vi "unified-2CAM.VI"() -> ()   [LabVIEW 2015]
uses:
  board.vis/Globals.vi
  <vilib>/Analysis/NI_AALBase.lvlib
panel:
  in  "send all":bool
  in  "Offset ADC 8":u16=49000
  in  "Offset ADC 3":u16=49000
  in  "Offset ADC 7":u16=49000
  in  "Offset ADC 2":u16=49000
  in  "Offset ADC 6":u16=49000
  in  "Offset ADC 1":u16=49000
  in  "Offset ADC 5":u16=49000
  in  "Offset ADC 4":u16=49000
  in  "custom pattern: 14bits (hex)":fxp<+,14,14>=100.0 format="%x"
  out "data adr  0x25":u16 format="%x"
  out "data adr  0x26":u16 format="%x"
  out "custom pattern: 14bits (dec)":fxp<+,14,14>
  in  "ADC mode":enum32{"1", "2", "3"}(radio)=enum."3"
  out "Signalverlaufgraph Cam 2":u16[](graph)=[100, 100, 100, 100, 100, 100, 100, 100, 100, 100, 100, 100, 100, 100, 100, 100, 100, 100, 100, 100, 100, 100, 100, 100, 100, 100, 100, 100, 100, 100, 100, 100, 100, 100, 100, 100, 100, 100, 100, 100, 100, 100, 100, 100, 100, 100, 100, 100, 100, 100, 100, 100, 100, 100, 100, 100, 100, 100, 100, 100, 100, 100, 100, 100, 100, 100, 100, 100, 100, 100, 100, 100, 100, 100, 100, 100, 100, 100, 100, 100, 100, 100, 100, 100, 100, 100, 100, 100, 100, 100, 100, 100, 100, 100, 100, 100, 100, 100, 100, 100, 100, 100, 100, 100, 100, 100, 100, 100, 100, 100, 100, 100, 100, 100, 100, 100, 100, 100, 100, 100, 100, 100, 100, 100, 100, 100, 100, 100, 100, 100, 100, 100, 100, 100, 100, 100, 100, 100, 100, 100, 100, 100, 100, 100, 100, 100, 100, 100, 100, 100, 100, 100, 100, 100, 100, 100, 100, 100, 100, 100, 100, 100, 100, 100, 100, 100, 100, 100, 100, 100, 100, 100, 100, 100, 100, 100, 100, 100, 100, 100, 100, 100, 100, 100, 100, 100, 100, 100, 100, 100, 100, 100, 100, 100, 100, 100, 100, 100, 100, 100, 100, 100, 100, 100, 100, 100, 100, 100, 100, 100, 100, 100, 100, 100, 100, 100, 100, 100, 100, 100, 100, 100, 100, 100, 100, 100, 100, 100, 100, 100, 100, 100, 100, 100, 100, 100, 100, 100, 100, 100, 100, 100, 100, 100, 100, 100, 100, 100, 100, 100, 100, 100, 100, 100, 100, 100, 100, 100, 100, 100, 100, 100, 100, 100, 100, 100, 100, 100, 100, 100, 100, 100, 100, 100, 100, 100, 100, 100, 100, 100, 100, 100, 100, 100, 100, 100, 100, 100, 100, 100, 100, 100, 100, 100, 100, 100, 100, 100, 100, 100, 100, 100, 100, 100, 100, 100, 100, 100, 100, 100, 100, 100, 100, 100, 100, 100, 100, 100, 100, 100, 100, 100, 100, 100, 100, 100, 100, 100, 100, 100, 100, 100, 100, 100, 100, 100, 100, 100, 100, 100, 100, 100, 100, 100, 100, 100, 100, 100, 100, 100, 100, 100, 100, 100, 100, 100, 100, 100, 100, 100, 100, 100, 100, 100, 100, 100, 100, 100, 100, 100, 100, 100, 100, 100, 100, 100, 100, 100, 100, 100, 100, 100, 100, 100, 100, 100, 100, 100, 100, 100, 100, 100, 100, 100, 100, 100, 100, 100, 100, 100, 100, 100, 100, 100, 100, 100, 100, 100, 100, 100, 100, 100, 100, 100, 100, 100, 100, 100, 100, 100, 100, 100, 100, 100, 100, 100, 100, 100, 100, 100, 100, 100, 100, 100, 100, 100, 100, 100, 100, 100, 100, 100, 100, 100, 100, 100, 100, 100, 100, 100, 100, 100, 100, 100, 100, 100, 100, 100, 100, 100, 100, 100, 100, 100, 100, 100, 100, 100, 100, 100, 100, 100, 100, 100, 100, 100, 100, 100, 100, 100, 100, 100, 100, 100, 100, 100, 100, 100, 100, 100, 100, 100, 100, 100, 100, 100, 100, 100, 100, 100, 100, 100, 100, 100, 100, 100, 100, 100, 100, 100, 100, 100, 100, 100, 100, 100, 100, 100, 100, 100, 100, 100, 100, 100, 100, 100, 100, 100, 100, 100, 100, 100, 100, 100, 100, 100, 100, 100, 100, 100, 100, 100, 100, 100, 100, 100, 100, 100, 100, 100, 100, 100, 100, 100, 100, 100, 100, 100, 100, 100, 100, 100, 100, 100, 100, 100, 100, 100, 100, 100, 100, 100, 100, 100, 100, 100, 100, 100, 100, 100, 100, 100, 100, 100, 100, 100, 100, 100, 100, 100, 100, 100, 100, 100, 100, 100, 100, 100, 100, 100, 100, 100, 100, 100, 100, 100, 100, 100, 100, 100, 100, 100, 100, 100, 100, 100, 100, 100, 100, 100, 100, 100, 100, 100, 100, 100, 100, 100, 100, 100, 100, 100, 100, 100, 100, 100, 100, 100, 100, 100, 100, 100, 100, 100, 100, 100, 100, 100, 100, 100, 100, 100, 100, 100, 100, 100, 100, 100, 100, 100, 100, 100, 100, 100, 100, 100, 100, 100, 100, 100, 100, 100, 100, 100, 100, 100, 100, 100, 100, 100, 100, 100, 100, 100, 100, 100, 100, 100, 100, 100, 100, 100, 100, 100, 100, 100, 100, 100, 100, 100, 100, 100, 100, 100, 100, 100, 100, 100, 100, 100, 100, 100, 100, 100, 100, 100, 100, 100, 100, 100, 100, 100, 100, 100, 100, 100, 100, 100, 100, 100, 100, 100, 100, 100, 100, 100, 100, 100, 100, 100, 100, 100, 100, 100, 100, 100, 100, 100, 100, 100, 100, 100, 100, 100, 100, 100, 100, 100, 100, 100, 100, 100, 100, 100, 100, 100, 100, 100, 100, 100, 100, 100, 100, 100, 100, 100, 100, 100, 100, 100, 100, 100, 100, 100, 100, 100, 100, 100, 100, 100, 100, 100, 100, 100, 100, 100, 100, 100, 100, 100, 100, 100, 100, 100, 100, 100, 100, 100, 100, 100, 100, 100, 100, 100, 100, 100, 100, 100, 100, 100, 100, 100, 100, 100, 100, 100, 100, 100, 100, 100, 100, 100, 100, 100, 100, 100, 100, 100, 100, 100, 100, 100, 100, 100, 100, 100, 100, 100, 100, 100, 100, 100, 100, 100, 100, 100, 100, 100, 100, 100, 100, 100, 100, 100, 100, 100, 100, 100, 100, 100, 100, 100, 100, 100, 100, 100, 100, 100, 100, 100, 100, 100, 100, 100, 100, 100, 100, 100, 100, 100, 100, 100, 100, 100, 100, 100, 100, 100, 100, 100, 100, 100, 100, 100, 100, 100, 100, 100, 100, 100, 100, 100, 100, 100, 100, 100, 100, 100, 100, 100, 100, 100, 100, 100, 100, 100, 100, 100, 100, 100, 100, 100, 100, 100, 100, 100, 100, 100, 100, 100, 100, 100, 100, 100, 100, 100, 100, 100, 100, 100, 100, 100, 100, 100, 100, 100, 100, 100, 100, 100, 100, 100, 100, 100, 100, 100, 100, 100, 100, 100, 100, 100, 100, 100, 100, 100, 100, 100, 100, 100, 100, 100, 100, 100, 100, 100, 100, 100, 100, 100, 100, 100, 100, 100, 100, 100, 100, 100, 100, 100, 100, 100, 100, 100, 100, 100, 100, 100, 100, 100, 100, 100, 100, 100, 100, 100, 100, 100, 100, 100, 100, 100, 100, 100, 100, 100, 100, 100, 100, 100, 100, 100, 100, 100, 100, 100, 100, 100, 100, 100, 100, 100, 100, 100, 100, 100, 100, 100, 100, 100, 100, 100, 100, 100, 100, 100, 100, 100, 100, 100, 100, 100, 100, 100, 100, 100, 100, 100, 100, 100, 100, 100, 100, 100, 100, 100, 100, 100, 100, 100, 100, 100, 100, 100, 100, 100, 100, 100]
  in  "extTrig":bool
  in  "ext. trig. slope":enum32{"1", "2", "3"}(radio)
  out "tRMS":dbl format="%0#.1f"
  out "mean":dbl=100.0 format="%#_4f"
  in  "rms_pixel":u16=100
  in  "is FFT":bool=TRUE
  in  "IR gain":bool
  in  "continuous":bool
  out "curr.block":u8=4
  out "Measure ON":bool
  in  "Board select\n1: board 1\n2: board 2\n3: both boards":u8=3
  in  "no.of blocks (nob)\npress enter":u32=4
  in  "block":u32(slide)=2 max=10 scale=0.9..4.0
  out "Signalverlaufgraph Board 2":u16[](graph)=[0, 0, 543, 543, 0, 1, 0, 0, 2, 2, 3, 3, 4, 4, 5, 5, 6, 6, 7, 7, 8, 8, 9, 9, 10, 10, 11, 11, 12, 12, 13, 13, 14, 14, 15, 15, 16, 16, 17, 17, 18, 18, 19, 19, 20, 20, 21, 21, 22, 22, 23, 23, 24, 24, 25, 25, 26, 26, 27, 27, 28, 28, 29, 29, 30, 30, 31, 31, 32, 32, 33, 33, 34, 34, 35, 35, 36, 36, 37, 37, 38, 38, 39, 39, 40, 40, 41, 41, 42, 42, 43, 43, 44, 44, 45, 45, 46, 46, 47, 47, 48, 48, 49, 49, 50, 50, 51, 51, 52, 52, 53, 53, 54, 54, 55, 55, 56, 56, 57, 57, 58, 58, 59, 59, 60, 60, 61, 61, 62, 62, 63, 63, 64, 64, 65, 65, 66, 66, 67, 67, 68, 68, 69, 69, 70, 70, 71, 71, 72, 72, 73, 73, 74, 74, 75, 75, 76, 76, 77, 77, 78, 78, 79, 79, 80, 80, 81, 81, 82, 82, 83, 83, 84, 84, 85, 85, 86, 86, 87, 87, 88, 88, 89, 89, 90, 90, 91, 91, 92, 92, 93, 93, 94, 94, 95, 95, 96, 96, 97, 97, 98, 98, 99, 99, 100, 100, 101, 101, 102, 102, 103, 103, 104, 104, 105, 105, 106, 106, 107, 107, 108, 108, 109, 109, 110, 110, 111, 111, 112, 112, 113, 113, 114, 114, 115, 115, 116, 116, 117, 117, 118, 118, 119, 119, 120, 120, 121, 121, 122, 122, 123, 123, 124, 124, 125, 125, 126, 126, 127, 127, 128, 128, 129, 129, 130, 130, 131, 131, 132, 132, 133, 133, 134, 134, 135, 135, 136, 136, 137, 137, 138, 138, 139, 139, 140, 140, 141, 141, 142, 142, 143, 143, 144, 144, 145, 145, 146, 146, 147, 147, 148, 148, 149, 149, 150, 150, 151, 151, 152, 152, 153, 153, 154, 154, 155, 155, 156, 156, 157, 157, 158, 158, 159, 159, 160, 160, 161, 161, 162, 162, 163, 163, 164, 164, 165, 165, 166, 166, 167, 167, 168, 168, 169, 169, 170, 170, 171, 171, 172, 172, 173, 173, 174, 174, 175, 175, 176, 176, 177, 177, 178, 178, 179, 179, 180, 180, 181, 181, 182, 182, 183, 183, 184, 184, 185, 185, 186, 186, 187, 187, 188, 188, 189, 189, 190, 190, 191, 191, 192, 192, 193, 193, 194, 194, 195, 195, 196, 196, 197, 197, 198, 198, 199, 199, 200, 200, 201, 201, 202, 202, 203, 203, 204, 204, 205, 205, 206, 206, 207, 207, 208, 208, 209, 209, 210, 210, 211, 211, 212, 212, 213, 213, 214, 214, 215, 215, 216, 216, 217, 217, 218, 218, 219, 219, 220, 220, 221, 221, 222, 222, 223, 223, 224, 224, 225, 225, 226, 226, 227, 227, 228, 228, 229, 229, 230, 230, 231, 231, 232, 232, 233, 233, 234, 234, 235, 235, 236, 236, 237, 237, 238, 238, 239, 239, 240, 240, 241, 241, 242, 242, 243, 243, 244, 244, 245, 245, 246, 246, 247, 247, 248, 248, 249, 249, 250, 250, 251, 251, 252, 252, 253, 253, 254, 254, 255, 255, 256, 256, 257, 257, 258, 258, 259, 259, 260, 260, 261, 261, 262, 262, 263, 263, 264, 264, 265, 265, 266, 266, 267, 267, 268, 268, 269, 269, 270, 270, 271, 271, 272, 272, 273, 273, 274, 274, 275, 275, 276, 276, 277, 277, 278, 278, 279, 279, 280, 280, 281, 281, 282, 282, 283, 283, 284, 284, 285, 285, 286, 286, 287, 287, 288, 288, 289, 289, 290, 290, 291, 291, 292, 292, 293, 293, 294, 294, 295, 295, 296, 296, 297, 297, 298, 298, 299, 299, 300, 300, 301, 301, 302, 302, 303, 303, 304, 304, 305, 305, 306, 306, 307, 307, 308, 308, 309, 309, 310, 310, 311, 311, 312, 312, 313, 313, 314, 314, 315, 315, 316, 316, 317, 317, 318, 318, 319, 319, 320, 320, 321, 321, 322, 322, 323, 323, 324, 324, 325, 325, 326, 326, 327, 327, 328, 328, 329, 329, 330, 330, 331, 331, 332, 332, 333, 333, 334, 334, 335, 335, 336, 336, 337, 337, 338, 338, 339, 339, 340, 340, 341, 341, 342, 342, 343, 343, 344, 344, 345, 345, 346, 346, 347, 347, 348, 348, 349, 349, 350, 350, 351, 351, 352, 352, 353, 353, 354, 354, 355, 355, 356, 356, 357, 357, 358, 358, 359, 359, 360, 360, 361, 361, 362, 362, 363, 363, 364, 364, 365, 365, 366, 366, 367, 367, 368, 368, 369, 369, 370, 370, 371, 371, 372, 372, 373, 373, 374, 374, 375, 375, 376, 376, 377, 377, 378, 378, 379, 379, 380, 380, 381, 381, 382, 382, 383, 383, 384, 384, 385, 385, 386, 386, 387, 387, 388, 388, 389, 389, 390, 390, 391, 391, 392, 392, 393, 393, 394, 394, 395, 395, 396, 396, 397, 397, 398, 398, 399, 399, 400, 400, 401, 401, 402, 402, 403, 403, 404, 404, 405, 405, 406, 406, 407, 407, 408, 408, 409, 409, 410, 410, 411, 411, 412, 412, 413, 413, 414, 414, 415, 415, 416, 416, 417, 417, 418, 418, 419, 419, 420, 420, 421, 421, 422, 422, 423, 423, 424, 424, 425, 425, 426, 426, 427, 427, 428, 428, 429, 429, 430, 430, 431, 431, 432, 432, 433, 433, 434, 434, 435, 435, 436, 436, 437, 437, 438, 438, 439, 439, 440, 440, 441, 441, 442, 442, 443, 443, 444, 444, 445, 445, 446, 446, 447, 447, 448, 448, 449, 449, 450, 450, 451, 451, 452, 452, 453, 453, 454, 454, 455, 455, 456, 456, 457, 457, 458, 458, 459, 459, 460, 460, 461, 461, 462, 462, 463, 463, 464, 464, 465, 465, 466, 466, 467, 467, 468, 468, 469, 469, 470, 470, 471, 471, 472, 472, 473, 473, 474, 474, 475, 475, 476, 476, 477, 477, 478, 478, 479, 479, 480, 480, 481, 481, 482, 482, 483, 483, 484, 484, 485, 485, 486, 486, 487, 487, 488, 488, 489, 489, 490, 490, 491, 491, 492, 492, 493, 493, 494, 494, 495, 495, 496, 496, 497, 497, 498, 498, 499, 499, 500, 500, 501, 501, 502, 502, 503, 503, 504, 504, 505, 505, 506, 506, 507, 507, 508, 508, 509, 509, 510, 510, 511, 511, 512, 512, 513, 513, 514, 514, 515, 515, 516, 516, 517, 517, 518, 518, 519, 519, 520, 520, 521, 521, 522, 522, 523, 523, 524, 524, 525, 525, 526, 526, 527, 527, 528, 528, 529, 529, 530, 530, 531, 531, 532, 532, 533, 533, 534, 534, 535, 535, 536, 536, 537, 537, 538, 538, 539, 539, 540, 540, 541, 541]
  out "Signalverlaufgraph":u16[](graph)=[542, 542, 543, 543, 49152, 2, 0, 566, 2, 2, 3, 3, 4, 4, 5, 5, 6, 6, 7, 7, 8, 8, 9, 9, 10, 10, 11, 11, 12, 12, 13, 13, 14, 14, 15, 15, 16, 16, 17, 17, 18, 18, 19, 19, 20, 20, 21, 21, 22, 22, 23, 23, 24, 24, 25, 25, 26, 26, 27, 27, 28, 28, 29, 29, 30, 30, 31, 31, 32, 32, 33, 33, 34, 34, 35, 35, 36, 36, 37, 37, 38, 38, 39, 39, 40, 40, 41, 41, 42, 42, 43, 43, 44, 44, 45, 45, 46, 46, 47, 47, 48, 48, 49, 49, 50, 50, 51, 51, 52, 52, 53, 53, 54, 54, 55, 55, 56, 56, 57, 57, 58, 58, 59, 59, 60, 60, 61, 61, 62, 62, 63, 63, 64, 64, 65, 65, 66, 66, 67, 67, 68, 68, 69, 69, 70, 70, 71, 71, 72, 72, 73, 73, 74, 74, 75, 75, 76, 76, 77, 77, 78, 78, 79, 79, 80, 80, 81, 81, 82, 82, 83, 83, 84, 84, 85, 85, 86, 86, 87, 87, 88, 88, 89, 89, 90, 90, 91, 91, 92, 92, 93, 93, 94, 94, 95, 95, 96, 96, 97, 97, 98, 98, 99, 99, 100, 100, 101, 101, 102, 102, 103, 103, 104, 104, 105, 105, 106, 106, 107, 107, 108, 108, 109, 109, 110, 110, 111, 111, 112, 112, 113, 113, 114, 114, 115, 115, 116, 116, 117, 117, 118, 118, 119, 119, 120, 120, 121, 121, 122, 122, 123, 123, 124, 124, 125, 125, 126, 126, 127, 127, 128, 128, 129, 129, 130, 130, 131, 131, 132, 132, 133, 133, 134, 134, 135, 135, 136, 136, 137, 137, 138, 138, 139, 139, 140, 140, 141, 141, 142, 142, 143, 143, 144, 144, 145, 145, 146, 146, 147, 147, 148, 148, 149, 149, 150, 150, 151, 151, 152, 152, 153, 153, 154, 154, 155, 155, 156, 156, 157, 157, 158, 158, 159, 159, 160, 160, 161, 161, 162, 162, 163, 163, 164, 164, 165, 165, 166, 166, 167, 167, 168, 168, 169, 169, 170, 170, 171, 171, 172, 172, 173, 173, 174, 174, 175, 175, 176, 176, 177, 177, 178, 178, 179, 179, 180, 180, 181, 181, 182, 182, 183, 183, 184, 184, 185, 185, 186, 186, 187, 187, 188, 188, 189, 189, 190, 190, 191, 191, 192, 192, 193, 193, 194, 194, 195, 195, 196, 196, 197, 197, 198, 198, 199, 199, 200, 200, 201, 201, 202, 202, 203, 203, 204, 204, 205, 205, 206, 206, 207, 207, 208, 208, 209, 209, 210, 210, 211, 211, 212, 212, 213, 213, 214, 214, 215, 215, 216, 216, 217, 217, 218, 218, 219, 219, 220, 220, 221, 221, 222, 222, 223, 223, 224, 224, 225, 225, 226, 226, 227, 227, 228, 228, 229, 229, 230, 230, 231, 231, 232, 232, 233, 233, 234, 234, 235, 235, 236, 236, 237, 237, 238, 238, 239, 239, 240, 240, 241, 241, 242, 242, 243, 243, 244, 244, 245, 245, 246, 246, 247, 247, 248, 248, 249, 249, 250, 250, 251, 251, 252, 252, 253, 253, 254, 254, 255, 255, 256, 256, 257, 257, 258, 258, 259, 259, 260, 260, 261, 261, 262, 262, 263, 263, 264, 264, 265, 265, 266, 266, 267, 267, 268, 268, 269, 269, 270, 270, 271, 271, 272, 272, 273, 273, 274, 274, 275, 275, 276, 276, 277, 277, 278, 278, 279, 279, 280, 280, 281, 281, 282, 282, 283, 283, 284, 284, 285, 285, 286, 286, 287, 287, 288, 288, 289, 289, 290, 290, 291, 291, 292, 292, 293, 293, 294, 294, 295, 295, 296, 296, 297, 297, 298, 298, 299, 299, 300, 300, 301, 301, 302, 302, 303, 303, 304, 304, 305, 305, 306, 306, 307, 307, 308, 308, 309, 309, 310, 310, 311, 311, 312, 312, 313, 313, 314, 314, 315, 315, 316, 316, 317, 317, 318, 318, 319, 319, 320, 320, 321, 321, 322, 322, 323, 323, 324, 324, 325, 325, 326, 326, 327, 327, 328, 328, 329, 329, 330, 330, 331, 331, 332, 332, 333, 333, 334, 334, 335, 335, 336, 336, 337, 337, 338, 338, 339, 339, 340, 340, 341, 341, 342, 342, 343, 343, 344, 344, 345, 345, 346, 346, 347, 347, 348, 348, 349, 349, 350, 350, 351, 351, 352, 352, 353, 353, 354, 354, 355, 355, 356, 356, 357, 357, 358, 358, 359, 359, 360, 360, 361, 361, 362, 362, 363, 363, 364, 364, 365, 365, 366, 366, 367, 367, 368, 368, 369, 369, 370, 370, 371, 371, 372, 372, 373, 373, 374, 374, 375, 375, 376, 376, 377, 377, 378, 378, 379, 379, 380, 380, 381, 381, 382, 382, 383, 383, 384, 384, 385, 385, 386, 386, 387, 387, 388, 388, 389, 389, 390, 390, 391, 391, 392, 392, 393, 393, 394, 394, 395, 395, 396, 396, 397, 397, 398, 398, 399, 399, 400, 400, 401, 401, 402, 402, 403, 403, 404, 404, 405, 405, 406, 406, 407, 407, 408, 408, 409, 409, 410, 410, 411, 411, 412, 412, 413, 413, 414, 414, 415, 415, 416, 416, 417, 417, 418, 418, 419, 419, 420, 420, 421, 421, 422, 422, 423, 423, 424, 424, 425, 425, 426, 426, 427, 427, 428, 428, 429, 429, 430, 430, 431, 431, 432, 432, 433, 433, 434, 434, 435, 435, 436, 436, 437, 437, 438, 438, 439, 439, 440, 440, 441, 441, 442, 442, 443, 443, 444, 444, 445, 445, 446, 446, 447, 447, 448, 448, 449, 449, 450, 450, 451, 451, 452, 452, 453, 453, 454, 454, 455, 455, 456, 456, 457, 457, 458, 458, 459, 459, 460, 460, 461, 461, 462, 462, 463, 463, 464, 464, 465, 465, 466, 466, 467, 467, 468, 468, 469, 469, 470, 470, 471, 471, 472, 472, 473, 473, 474, 474, 475, 475, 476, 476, 477, 477, 478, 478, 479, 479, 480, 480, 481, 481, 482, 482, 483, 483, 484, 484, 485, 485, 486, 486, 487, 487, 488, 488, 489, 489, 490, 490, 491, 491, 492, 492, 493, 493, 494, 494, 495, 495, 496, 496, 497, 497, 498, 498, 499, 499, 500, 500, 501, 501, 502, 502, 503, 503, 504, 504, 505, 505, 506, 506, 507, 507, 508, 508, 509, 509, 510, 510, 511, 511, 512, 512, 513, 513, 514, 514, 515, 515, 516, 516, 517, 517, 518, 518, 519, 519, 520, 520, 521, 521, 522, 522, 523, 523, 524, 524, 525, 525, 526, 526, 527, 527, 528, 528, 529, 529, 530, 530, 531, 531, 532, 532, 533, 533, 534, 534, 535, 535, 536, 536, 537, 537, 538, 538, 539, 539, 540, 540, 541, 541]
  out "boards recognised":u8=1
  in  "alloc mem":bool
  out "FREE \nRAM MB":dbl=16168.06640625
  out "BUILT-IN\nRAM MB":dbl=18096.171875
  out "SEC":dbl=4.4
  out "MB RAM":dbl=9.130859375
  in  "DAT in 10ns":u32
  in  "stop all":bool
  in  "start":bool
  in  "sample":u32(slide)=567 max=3000 scale=0.9..1100.0
  in  "no.of samples (nos)":u32=1100
  in  "exposuretime[ms]":dbl=0.1 format="%.3f"
  # "press Esc to stop measurement"
  # "exit here"
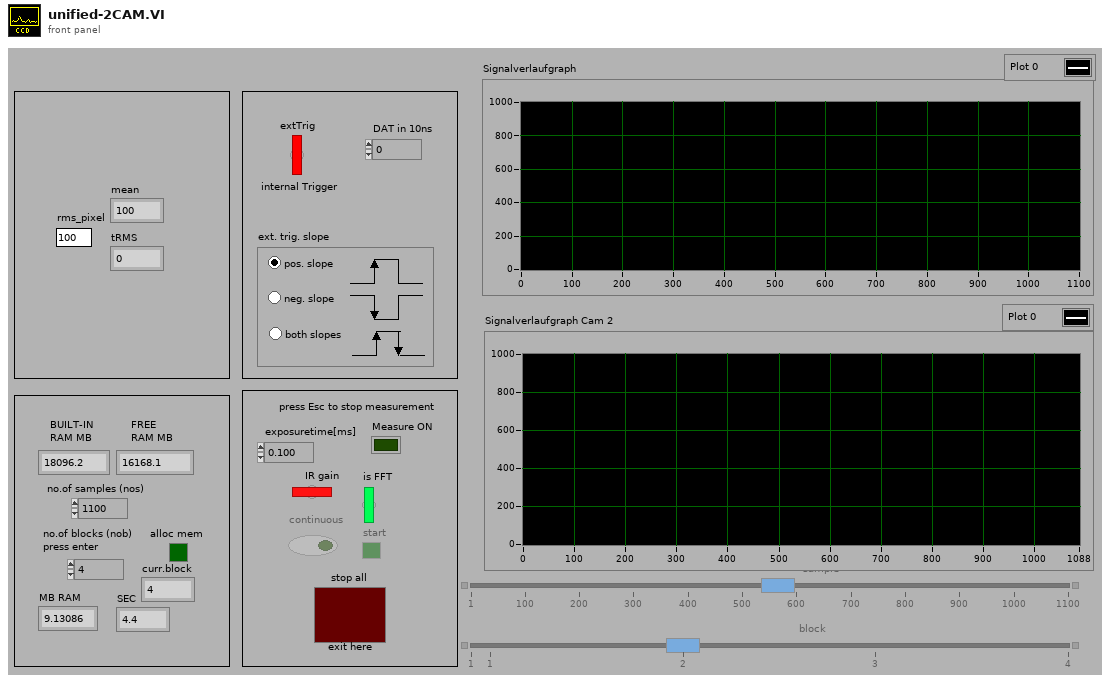
[diagram p1: front panel]
types:
  T1 = enum8{"Enabled", "Disabled", "Disabled and Grayed Out"}
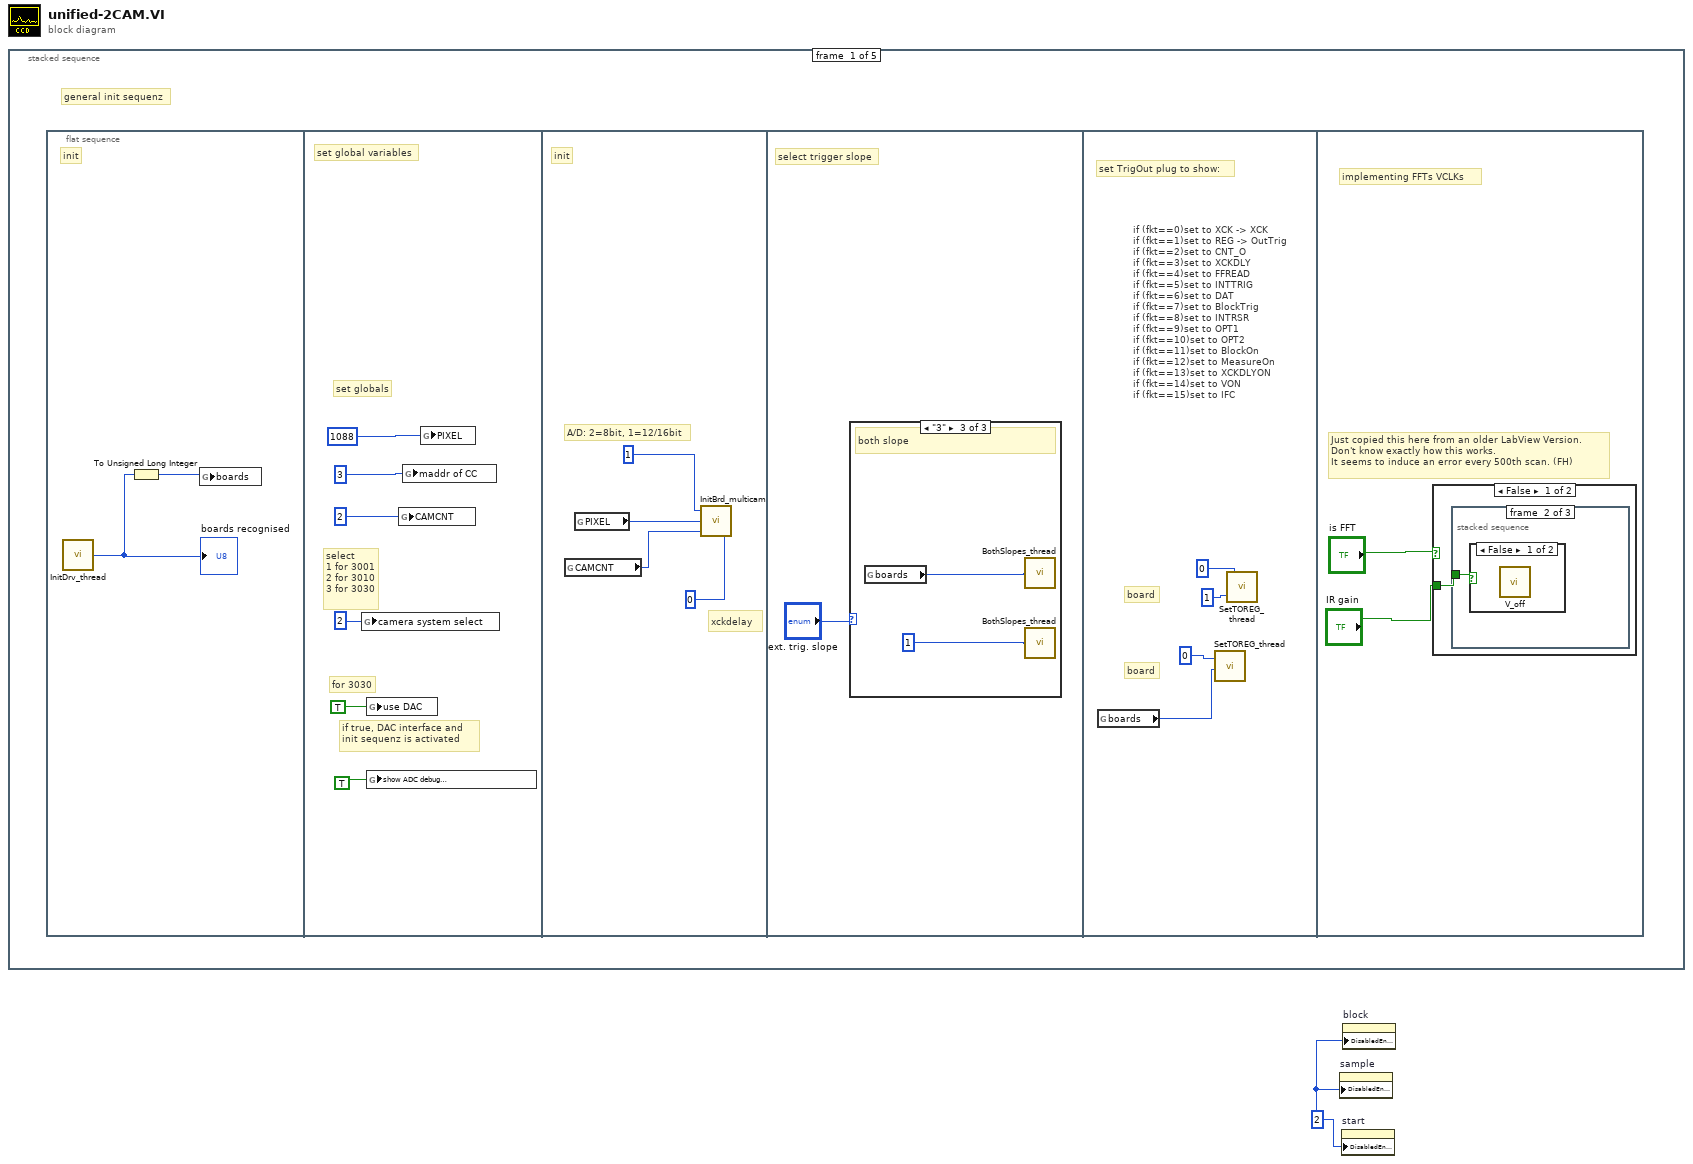
[diagram p0: block diagram]
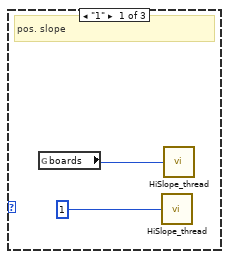
[diagram p2: hidden frame]
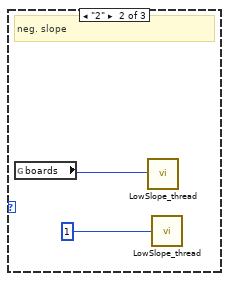
[diagram p3: hidden frame]
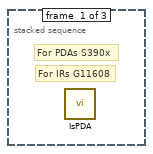
[diagram p4: hidden frame]
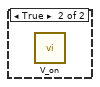
[diagram p5: hidden frame]
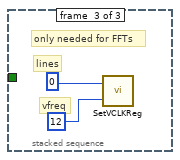
[diagram p6: hidden frame]
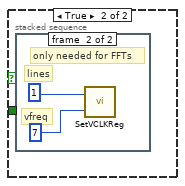
[diagram p7: hidden frame]
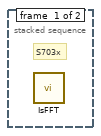
[diagram p8: hidden frame]
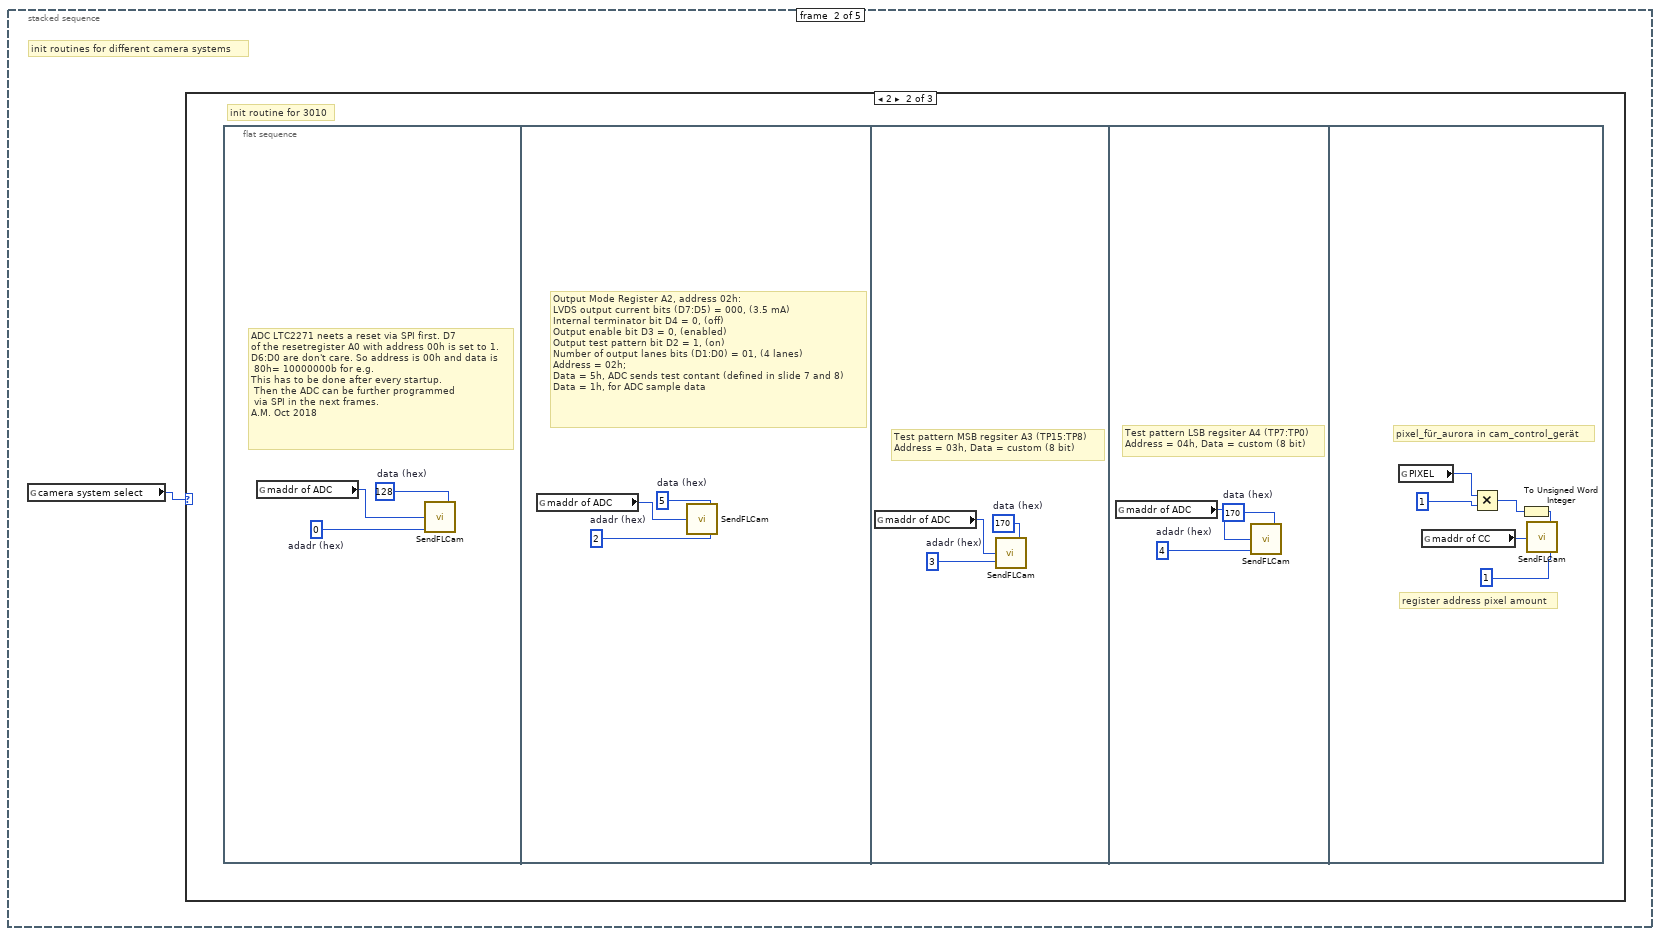
[diagram p9: hidden frame]
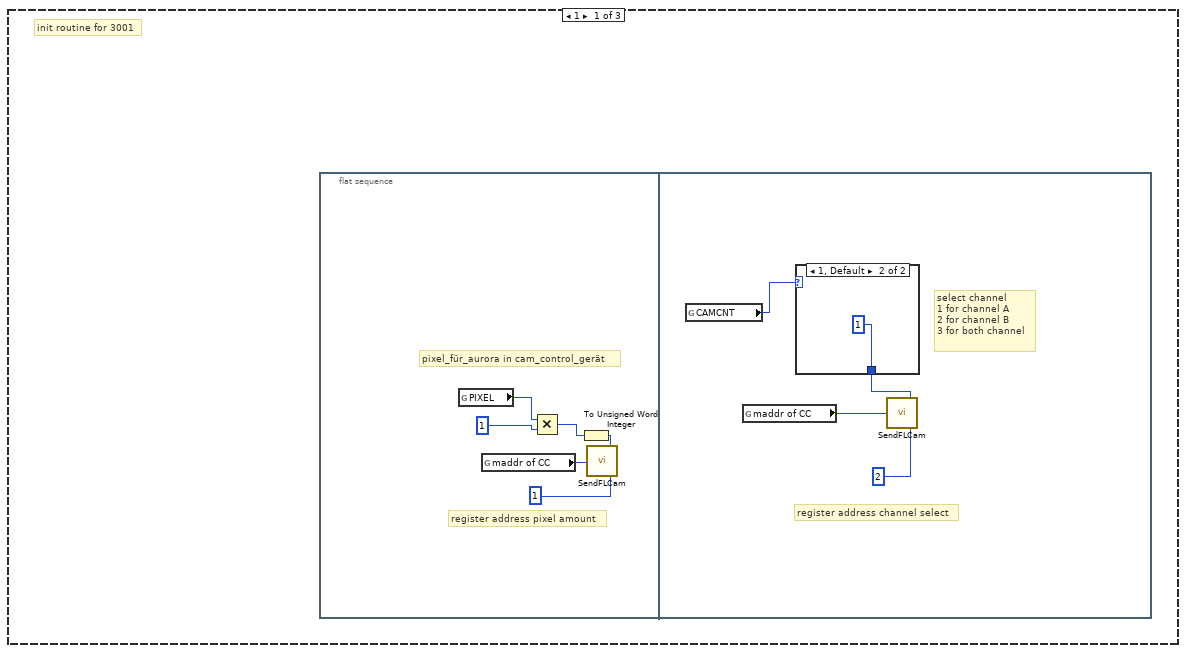
[diagram p10: hidden frame]
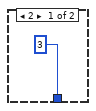
[diagram p11: hidden frame]
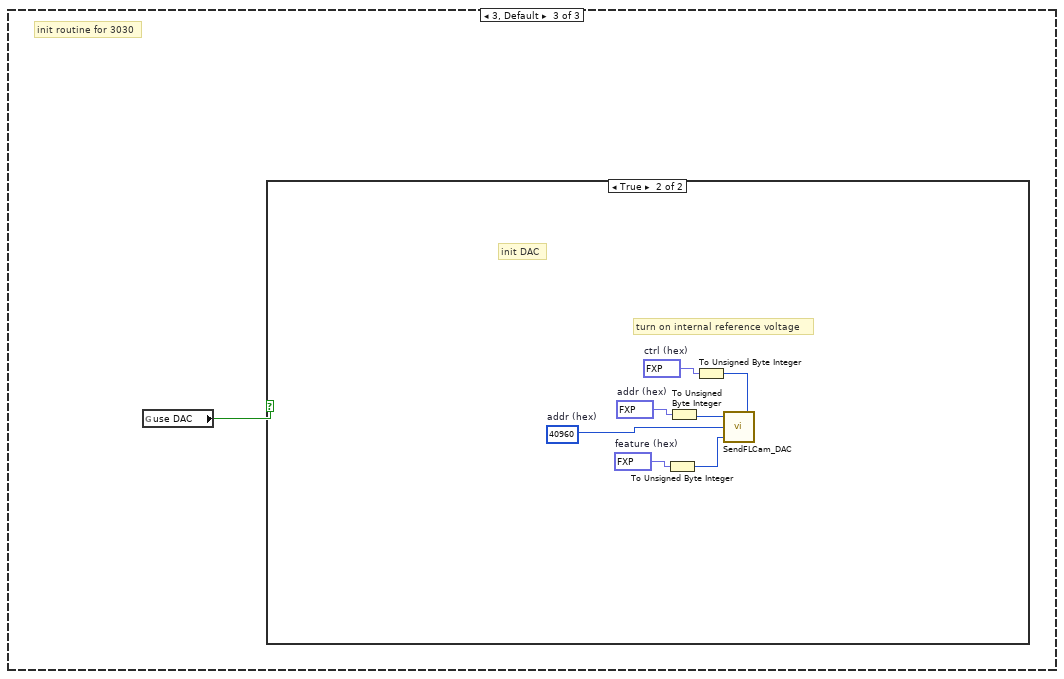
[diagram p12: hidden frame]
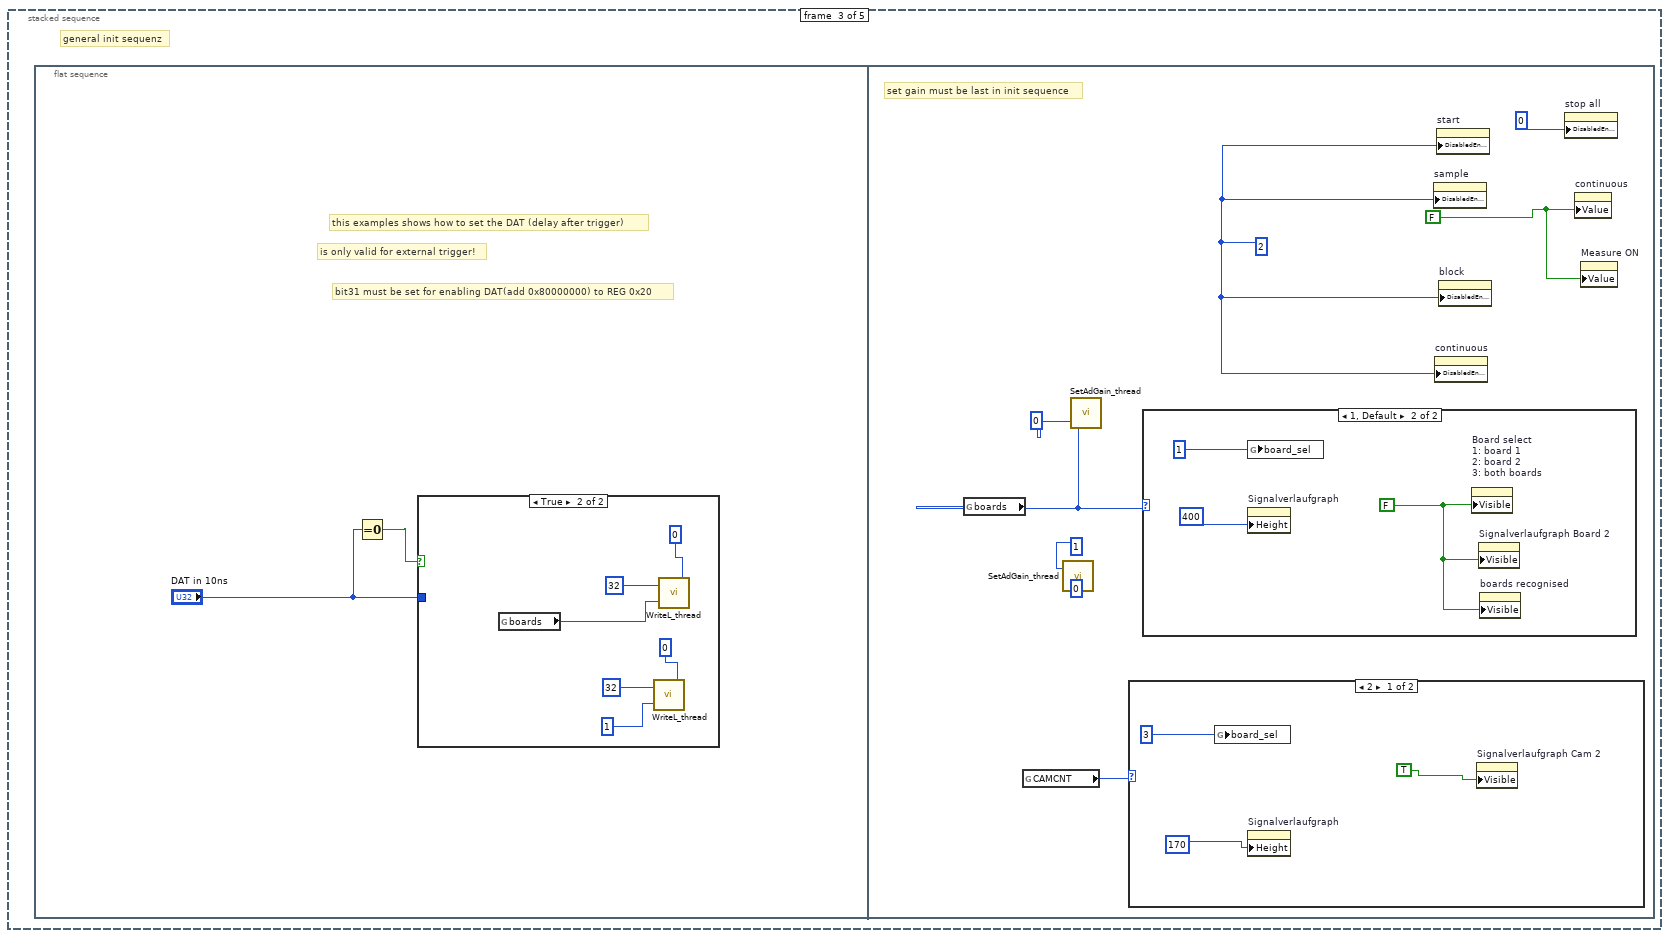
[diagram p14: hidden frame]
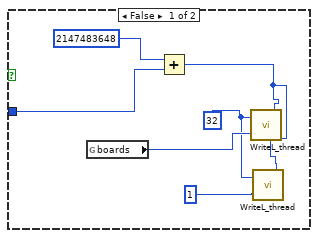
[diagram p15: hidden frame]
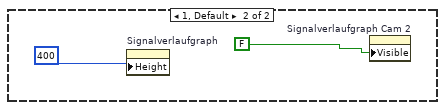
[diagram p16: hidden frame]
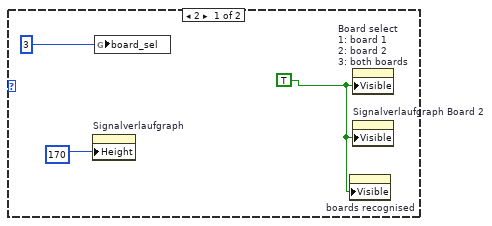
[diagram p17: hidden frame]
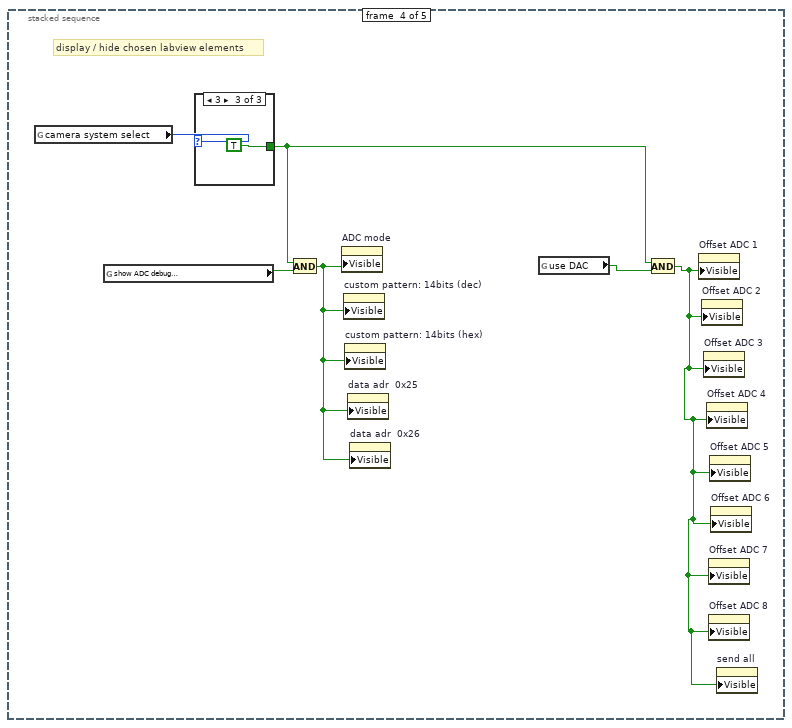
[diagram p18: hidden frame]
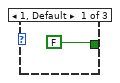
[diagram p19: hidden frame]
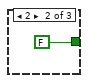
[diagram p20: hidden frame]
diagram:
  w1 = 2
  n1 = stacked-sequence {
    frame #0 {
      # "general init sequenz"
      n2 = flat-sequence {
        frame #0 {
          # "init"
          n3 = call "InitDrv_thread.vi"() -> ("Boards"=w2:u8)  [unwired: 1 in]
          "boards recognised" <- w2
          n4 = To Unsigned Long Integer(number=w2) -> (unsigned 32bit integer=w3:u32)
          n5 = global write "Globals.vi" "boards"(w3) -> ()
        }
        frame #1 {
          # "if true, DAC interface and \ninit sequenz is activated"
          # "for 3030"
          # "set global variables"
          # "select \n1 for 3001\n2 for 3010\n3 for 3030"
          # "set globals"
          n6 = global write "Globals.vi" "camera system select"(u8 2) -> ()
          n7 = global write "Globals.vi" "use DAC"(TRUE) -> ()
          n8 = global write "Globals.vi" "show ADC debug \ninterface"(TRUE) -> ()
          n9 = global write "Globals.vi" "CAMCNT"(u32 2) -> ()
          n10 = global write "Globals.vi" "maddr of CC"(u8 3) -> ()
          n11 = global write "Globals.vi" "PIXEL"(u32 1088) -> ()
        }
        frame #2 {
          # "init"
          # "xckdelay"
          # "A/D: 2=8bit, 1=12/16bit"
          n12 = global read "Globals.vi" "CAMCNT"() -> (w10:u32)
          n13 = global read "Globals.vi" "PIXEL"() -> (w13:u32)
          n14 = call "InitBrd_multicam.vi"("xckdly"=u32 0, "camcnt"=w10, "pixel"=w13, "flag816"=u32 1) -> ()  [unwired: 2 in]
        }
        frame #3 {
          # "select trigger slope"
          n15 = case shown="\"3\"" "ext. trig. slope" {
            frame "1" {
              # "pos. slope"
              n16 = global read "Globals.vi" "boards"() -> (w15:u32)
              n17 = call "HiSlope_thread.vi"("board"=u32 1) -> ()  [unwired: 1 in]
              n18 = call "HiSlope_thread.vi"("board"=w15) -> ()  [unwired: 1 in]
            }
            frame "2" {
              # "neg. slope"
              n19 = global read "Globals.vi" "boards"() -> (w18:u32)
              n20 = call "LowSlope_thread.vi"("board"=w18) -> ()  [unwired: 1 in]
              n21 = call "LowSlope_thread.vi"("board"=u32 1) -> ()  [unwired: 1 in]
            }
            frame "3" {
              # "both slope"
              n22 = global read "Globals.vi" "boards"() -> (w19:u32)
              n23 = call "BothSlopes_thread.vi"("board"=w19) -> ()  [unwired: 1 in]
              n24 = call "BothSlopes_thread.vi"("board"=u32 1) -> ()  [unwired: 1 in]
            }
          }
        }
        frame #4 {
          # "if (fkt==0)set to XCK -> XCK\nif (fkt==1)set to REG -> OutTrig\nif (fkt==2)set to CNT_O\nif (fkt==3)set to XCKDLY\nif (fkt==4)set to FFREAD\nif (fkt==5)set to INTTRIG\nif (fkt==6)set to DAT\nif (fkt==7)set to BlockTrig\nif (fkt==8)set to INTRSR\nif (fkt==9)set to OPT1\nif (fkt==10)set to OPT2\nif (fkt==11)set to BlockOn\nif (fkt==12)set to MeasureOn\nif (fkt==13)set to XCKDLYON \nif (fkt==14)set to VON         \nif (fkt==15)set to IFC"
          # "board"
          # "board"
          # "set TrigOut plug to show:"
          n25 = global read "Globals.vi" "boards"() -> (w24:u32)
          n26 = call "SetTOREG_thread.vi"("board"=w24, "fkt"=u8 0) -> ()  [unwired: 1 in]
          n27 = call "SetTOREG_thread.vi"("board"=u32 1, "fkt"=u8 0) -> ()  [unwired: 1 in]
        }
        frame #5 {
          # "implementing FFTs VCLKs"
          # "Just copied this here from an older LabView Version. \nDon't know exactly how this works.\nIt seems to induce an error every 500th scan. (FH)"
          n28 = case shown="False" "is FFT" {
            tunnel: "IR gain" -> [w27 _]
            frame False {
              n29 = stacked-sequence {
                tunnel: w27 -> [_ w28 _]
                frame #0 {
                  # "For IRs G11608"
                  # "For PDAs S390x"
                  n30 = call "IsPDA.vi"() -> ()  [unwired: 1 in]
                }
                frame #1 {
                  n31 = case shown="False" w28 {
                    frame False {
                      n32 = call "V_off.vi"() -> ()  [unwired: 1 in]
                    }
                    frame True {
                      n33 = call "V_on.vi"() -> ()  [unwired: 1 in]
                    }
                  }
                }
                frame #2 {
                  # "only needed for FFTs"
                  # "vfreq"
                  # "lines"
                  n34 = call "SetVCLKReg.vi"("vfreq"=u8 12, "lines"=u32 0) -> ()  [unwired: 1 in]
                }
              }
            }
            frame True {
              n35 = stacked-sequence {
                frame #0 {
                  # "S703x"
                  n36 = call "IsFFT.vi"() -> ()  [unwired: 1 in]
                }
                frame #1 {
                  # "only needed for FFTs"
                  # "vfreq"
                  # "lines"
                  n37 = call "SetVCLKReg.vi"("vfreq"=u8 7, "lines"=u32 1) -> ()  [unwired: 1 in]
                }
              }
            }
          }
        }
      }
    }
    frame #1 {
      # "init routines for different camera systems"
      n38 = global read "Globals.vi" "camera system select"() -> (w33:u8)
      n39 = case shown="2" w33 {
        frame 1 {
          # "init routine for 3001"
          n40 = flat-sequence {
            frame #0 {
              # "register address pixel amount"
              # "pixel_für_aurora in cam_control_gerät"
              n41 = global read "Globals.vi" "PIXEL"() -> (w38:u32)
              n42 = global read "Globals.vi" "maddr of CC"() -> (w35:u8)
              n43 = Multiply(x=w38, y=u32 1) -> (x*y=w37:u32)
              n44 = To Unsigned Word Integer(number=w37) -> (unsigned 16bit integer=w36:u16)
              n45 = call "SendFLCam.vi"("madr"=w35, "data"=w36, "adadr"=u8 1) -> ()
            }
            frame #1 {
              # "select channel\n1 for channel A\n2 for channel B\n3 for both channel"
              # "register address channel select"
              n46 = global read "Globals.vi" "CAMCNT"() -> (w41:u32)
              n47 = global read "Globals.vi" "maddr of CC"() -> (w43:u8)
              n48 = case shown="1, Default" w41 {
                tunnel: [u16 3 u16 1] -> w40
                frame 2 {
                }
                frame 1, Default {
                }
              }
              n49 = call "SendFLCam.vi"("madr"=w43, "data"=w40, "adadr"=u8 2) -> ()
            }
          }
        }
        frame 2 {
          # "init routine for 3010"
          n50 = flat-sequence {
            frame #0 {
              w48 = u16 128  # data (hex)
              w47 = u8 0  # adadr (hex)
              # "ADC LTC2271 neets a reset via SPI first. D7\nof the resetregister A0 with address 00h is set to 1.\nD6:D0 are don't care. So address is 00h and data is\n 80h= 10000000b for e.g.  \nThis has to be done after every startup.\n Then the ADC can be further programmed\n via SPI in the next frames.\nA.M. Oct 2018"
              n51 = global read "Globals.vi" "maddr of ADC"() -> (w46:u8)
              n52 = call "SendFLCam.vi"("madr"=w46, "data"=w48, "adadr"=w47) -> ()
            }
            frame #1 {
              w50 = u16 5  # data (hex)
              w51 = u8 2  # adadr (hex)
              # "Output Mode Register A2, address 02h:\nLVDS output current bits (D7:D5) = 000, (3.5 mA)\nInternal terminator bit D4 = 0, (off)\nOutput enable bit D3 = 0, (enabled)\nOutput test pattern bit D2 = 1, (on)\nNumber of output lanes bits (D1:D0) = 01, (4 lanes)\nAddress = 02h;\nData = 5h, ADC sends test contant (defined in slide 7 and 8)\nData = 1h, for ADC sample data"
              n53 = global read "Globals.vi" "maddr of ADC"() -> (w49:u8)
              n54 = call "SendFLCam.vi"("madr"=w49, "data"=w50, "adadr"=w51) -> ()
            }
            frame #2 {
              w53 = u16 170  # data (hex)
              w54 = u8 3  # adadr (hex)
              # "Test pattern MSB regsiter A3 (TP15:TP8)\nAddress = 03h, Data = custom (8 bit)"
              n55 = global read "Globals.vi" "maddr of ADC"() -> (w52:u8)
              n56 = call "SendFLCam.vi"("madr"=w52, "data"=w53, "adadr"=w54) -> ()
            }
            frame #3 {
              w56 = u16 170  # data (hex)
              w57 = u8 4  # adadr (hex)
              # "Test pattern LSB regsiter A4 (TP7:TP0)\nAddress = 04h, Data = custom (8 bit)"
              n57 = global read "Globals.vi" "maddr of ADC"() -> (w55:u8)
              n58 = call "SendFLCam.vi"("madr"=w55, "data"=w56, "adadr"=w57) -> ()
            }
            frame #4 {
              # "register address pixel amount"
              # "pixel_für_aurora in cam_control_gerät"
              n59 = global read "Globals.vi" "PIXEL"() -> (w62:u32)
              n60 = global read "Globals.vi" "maddr of CC"() -> (w59:u8)
              n61 = Multiply(x=w62, y=u32 1) -> (x*y=w61:u32)
              n62 = To Unsigned Word Integer(number=w61) -> (unsigned 16bit integer=w60:u16)
              n63 = call "SendFLCam.vi"("madr"=w59, "data"=w60, "adadr"=u8 1) -> ()
            }
          }
        }
        frame 3, Default {
          # "init routine for 3030"
          n64 = global read "Globals.vi" "use DAC"() -> (w64:bool)
          n65 = case shown="True" w64 {
            frame False {
            }
            frame True {
              w65 = u16 40960  # addr (hex)
              w68 = fxp<+,4,4> 0.0  # feature (hex)
              w69 = fxp<+,4,4> 0.0  # addr (hex)
              w71 = fxp<+,4,4> 9.0  # ctrl (hex)
              # "turn on internal reference voltage"
              # "init DAC"
              n66 = To Unsigned Byte Integer(number=w68) -> (unsigned 8bit integer=w67:u8)
              n67 = To Unsigned Byte Integer(number=w69) -> (unsigned 8bit integer=w66:u8)
              n68 = To Unsigned Byte Integer(number=w71) -> (unsigned 8bit integer=w70:u8)
              n69 = call "SendFLCam_DAC.vi"("ctrl"=w70, "feature"=w67, "data"=w65, "addr"=w66) -> ()
            }
          }
        }
      }
    }
    frame #2 {
      # "general init sequenz"
      n70 = flat-sequence {
        frame #0 {
          # "bit31 must be set for enabling DAT(add 0x80000000) to REG 0x20"
          # "is only valid for external trigger!"
          # "this examples shows how to set the DAT (delay after trigger)"
          n71 = Equal To 0?(x="DAT in 10ns") -> (x = 0?=w73:bool)
          n72 = case shown="True" w73 {
            tunnel: "DAT in 10ns" -> [w78 _]
            frame False {
              w75 = u32 32
              n73 = global read "Globals.vi" "boards"() -> (w77:u32)
              n74 = Add(x=u32 2147483648, y=w78) -> (x+y=w76:u32)
              n75 = call "WriteL_thread.vi"("val"=w76, "board"=w77, "offset"=w75) -> ()
              n76 = call "WriteL_thread.vi"("val"=w76, "board"=u32 1, "offset"=w75) -> ()
            }
            frame True {
              n77 = global read "Globals.vi" "boards"() -> (w84:u32)
              n78 = call "WriteL_thread.vi"("val"=u32 0, "board"=u32 1, "offset"=u32 32) -> ()
              n79 = call "WriteL_thread.vi"("val"=u32 0, "board"=w84, "offset"=u32 32) -> ()
            }
          }
        }
        frame #1 {
          w88 = FALSE
          w93 = 2
          # "set gain must be last in init sequence"
          n80 = global read "Globals.vi" "boards"() -> (w87:u32)
          n81 = global read "Globals.vi" "CAMCNT"() -> (w86:u32)
          n82 = call "SetAdGain_thread.vi"("gain"=u8 0, "board"=u32 1) -> ()  [unwired: 1 in]
          n83 = call "SetAdGain_thread.vi"("gain"=u8 0, "board"=w87) -> ()  [unwired: 1 in]
          n84 = case shown="2" w86 {
            frame 2 {
              n85 = global write "Globals.vi" "board_sel"(u8 3) -> ()
              n86 = property on="Signalverlaufgraph" class="WFGraph (strict)"("Height"=u8 170) -> ()  [unwired: 2 in, 2 out]
              n87 = property on="Signalverlaufgraph Cam 2" class="WFGraph (strict)"("Visible"=TRUE) -> ()  [unwired: 2 in, 2 out]
            }
            frame 1, Default {
              n88 = property on="Signalverlaufgraph" class="WFGraph (strict)"("Height"=400) -> ()  [unwired: 2 in, 2 out]
              n89 = property on="Signalverlaufgraph Cam 2" class="WFGraph (strict)"("Visible"=FALSE) -> ()  [unwired: 2 in, 2 out]
            }
          }
          n90 = case shown="1, Default" w87 {
            frame 2 {
              w101 = TRUE
              n91 = property on="Signalverlaufgraph" class="WFGraph (strict)"("Height"=u8 170) -> ()  [unwired: 2 in, 2 out]
              n92 = global write "Globals.vi" "board_sel"(u8 3) -> ()
              n93 = property on="boards recognised" class="DigNum (strict)"("Visible"=w101) -> ()  [unwired: 2 in, 2 out]
              n94 = property on="Board select\n1: board 1\n2: board 2\n3: both boards" class="DigNum (strict)"("Visible"=w101) -> ()  [unwired: 2 in, 2 out]
              n95 = property on="Signalverlaufgraph Board 2" class="WFGraph (strict)"("Visible"=w101) -> ()  [unwired: 2 in, 2 out]
            }
            frame 1, Default {
              w102 = FALSE
              n96 = global write "Globals.vi" "board_sel"(u8 1) -> ()
              n97 = property on="Signalverlaufgraph" class="WFGraph (strict)"("Height"=400) -> ()  [unwired: 2 in, 2 out]
              n98 = property on="Board select\n1: board 1\n2: board 2\n3: both boards" class="DigNum (strict)"("Visible"=w102) -> ()  [unwired: 2 in, 2 out]
              n99 = property on="Signalverlaufgraph Board 2" class="WFGraph (strict)"("Visible"=w102) -> ()  [unwired: 2 in, 2 out]
              n100 = property on="boards recognised" class="DigNum (strict)"("Visible"=w102) -> ()  [unwired: 2 in, 2 out]
            }
          }
          n101 = property on="sample" class="Slide (strict)"("DisabledEnum"=w93) -> ()  [unwired: 2 in, 2 out]
          n102 = property on="continuous" class="Bool (strict)"("DisabledEnum"=w93) -> ()  [unwired: 2 in, 2 out]
          n103 = property on="start" class="Bool (strict)"("DisabledEnum"=w93) -> ()  [unwired: 2 in, 2 out]
          n104 = property on="block" class="Slide (strict)"("DisabledEnum"=w93) -> ()  [unwired: 2 in, 2 out]
          n105 = property on="stop all" class="Bool (strict)"("DisabledEnum"=0) -> ()  [unwired: 2 in, 2 out]
          n106 = property on="continuous" class="Bool (strict)"("Value"=w88) -> ()  [unwired: 2 in, 2 out]
          n107 = property on="Measure ON" class="Bool (strict)"("Value"=w88) -> ()  [unwired: 2 in, 2 out]
        }
      }
    }
    frame #3 {
      # "display / hide chosen labview elements"
      n108 = global read "Globals.vi" "camera system select"() -> (w110:u8)
      n109 = global read "Globals.vi" "show ADC debug \ninterface"() -> (w108:bool)
      n110 = case shown="3" w110 {
        tunnel: [FALSE FALSE TRUE] -> w106
        frame 1, Default {
        }
        frame 2 {
        }
        frame 3 {
        }
      }
      n111 = And(x=w106, y=w108) -> (x .and. y?=w109:bool)
      n112 = property on="ADC mode" class="RadioBtnsControl (strict)"("Visible"=w109) -> ()  [unwired: 2 in, 2 out]
      n113 = property on="custom pattern: 14bits (dec)" class="DigNum (strict)"("Visible"=w109) -> ()  [unwired: 2 in, 2 out]
      n114 = property on="custom pattern: 14bits (hex)" class="DigNum (strict)"("Visible"=w109) -> ()  [unwired: 2 in, 2 out]
      n115 = property on="data adr  0x25" class="DigNum (strict)"("Visible"=w109) -> ()  [unwired: 2 in, 2 out]
      n116 = property on="data adr  0x26" class="DigNum (strict)"("Visible"=w109) -> ()  [unwired: 2 in, 2 out]
      n117 = global read "Globals.vi" "use DAC"() -> (w107:bool)
      n118 = And(x=w106, y=w107) -> (x .and. y?=w105:bool)
      n119 = property on="Offset ADC 1" class="DigNum (strict)"("Visible"=w105) -> ()  [unwired: 2 in, 2 out]
      n120 = property on="Offset ADC 2" class="DigNum (strict)"("Visible"=w105) -> ()  [unwired: 2 in, 2 out]
      n121 = property on="Offset ADC 3" class="DigNum (strict)"("Visible"=w105) -> ()  [unwired: 2 in, 2 out]
      n122 = property on="Offset ADC 4" class="DigNum (strict)"("Visible"=w105) -> ()  [unwired: 2 in, 2 out]
      n123 = property on="Offset ADC 7" class="DigNum (strict)"("Visible"=w105) -> ()  [unwired: 2 in, 2 out]
      n124 = property on="Offset ADC 8" class="DigNum (strict)"("Visible"=w105) -> ()  [unwired: 2 in, 2 out]
      n125 = property on="Offset ADC 5" class="DigNum (strict)"("Visible"=w105) -> ()  [unwired: 2 in, 2 out]
      n126 = property on="Offset ADC 6" class="DigNum (strict)"("Visible"=w105) -> ()  [unwired: 2 in, 2 out]
      n127 = property on="send all" class="Bool (strict)"("Visible"=w105) -> ()  [unwired: 2 in, 2 out]
    }
    frame #4 {
      # "event structure while running"
      n128 = while {
        stop <- w115 stop-if-true
        n129 = event shown="[19] \"send all\": Value Change" {
          selector: _ -> [_ _ _ _ _ _ _ _ _ _ _ _ _ _ _ _ _ _ _ _]
          dyn-events: _ -> [_ _ _ _ _ _ _ _ _ _ _ _ _ _ _ _ _ _ _ _]
          timeout: 100 -> [_ _ _ _ _ _ _ _ _ _ _ _ _ _ _ _ _ _ _ _]
          tunnel: [_ _ _ _ _ _ _ _ w242 _ _ _ _ _ _ _ _ _ _ _] -> w115
          event Timeout {
            # "only refresh the frames if measure on"
            # "compares measure on signal from hardware with measure on lamp\nwhen diffrent than write new measure on value to lamp"
            # "timout excecutes every 100ms"
            # "userinfo of RAM, MeasureOB, Curr.Block and setting display event in cont mode"
            n130 = event-data() -> ()  [unwired: 1 in, 3 out]
            n131 = call "ReadB.vi"("Offset"=u32 64) -> ("Data"=w132:u8)
            n132 = call "FreeMemInfo.vi"() -> ("PhysicalSpace"=→"BUILT-IN\nRAM MB":dbl, "PhysicalFreeSpace"=→"FREE \nRAM MB":dbl)  [unwired: 1 in]
            n133 = Number To Boolean Array(number=w132) -> (Boolean array=w131:bool[])
            n134 = property on="Measure ON" class="Bool (strict)"() -> ("Value"=w126:bool)  [unwired: 2 in, 2 out]
            n135 = Index Array(array=w131, index=5) -> (element=w122:bool)
            n136 = Not Equal?(x=w126, y=w122) -> (x != y?=w125:bool)
            n137 = case shown="True" w125 {
              tunnel: w122 -> [_ w136]
              frame False {
              }
              frame True {
                n138 = property on="Measure ON" class="Bool (strict)"("Val(Sgnl)"=w136) -> ()  [unwired: 2 in, 2 out]
              }
            }
            n139 = property on="continuous" class="Bool (strict)"() -> ("DisabledEnum"=w119:T1)  [unwired: 2 in, 2 out]
            n140 = property on="continuous" class="Bool (strict)"() -> ("Value"=w128:bool)  [unwired: 2 in, 2 out]
            n141 = To Unsigned Byte Integer(number=w119) -> (unsigned 8bit integer=w120:u8)
            n142 = Equal?(x=w120, y=u8 0) -> (x = y?=w127:bool)
            n143 = And(x=w128, y=w127) -> (x .and. y?=w124:bool)
            n144 = And(x=w124, y=w122) -> (x .and. y?=w123:bool)
            n145 = call "ReadB.vi"("Offset"=u32 88) -> ("Data"=w117:u8)
            n146 = global read "Globals.vi" "CAMCNT"() -> (w116:u32)
            n147 = case shown="True" w123 {
              frame False {
              }
              frame True {
                # "refresh RMS.\nMaybe this is not a good style.\nIt's not clear to me which values are \nincluded to RMS measurement.\nBetter would be a refresh when all\nblocks are done."
                # "trigger the \ndisplay event"
                n148 = property on="rms_pixel" class="DigNum (strict)"() -> ("Value"=w137:u16)  [unwired: 2 in, 2 out]
                n149 = property on="sample" class="Slide (strict)"() -> ("Value"=w138:u32)  [unwired: 2 in, 2 out]
                n150 = property on="sample" class="Slide (strict)"("Val(Sgnl)"=w138) -> ()  [unwired: 2 in, 2 out]
                n151 = property on="rms_pixel" class="DigNum (strict)"("Val(Sgnl)"=w137) -> ()  [unwired: 2 in, 2 out]
              }
            }
            n152 = Divide(x=w117, y=w116) -> (x/y=→"curr.block":dbl)
          }
          event "Measure ON": Value Change {
            # "triggers on value change of measure on. this happens on start of measurement and after measurement\nwhen continuous: not after finishing all blocks, only when exiting measurement"
            n153 = event-data() -> ("NewVal"=w139:bool)  [unwired: 1 in, 5 out]
            n154 = property on="continuous" class="Bool (strict)"() -> ("Value"=w140:bool)  [unwired: 2 in, 2 out]
            n155 = And(x=w140, y=w139) -> (x .and. y?=w141:bool)
            n156 = case shown="False" w139 {
              frame False {
                n157 = property on="stop all" class="Bool (strict)"("DisabledEnum"=0) -> ()  [unwired: 2 in, 2 out]
              }
              frame True {
              }
            }
            n158 = case shown="True" w141 {
              frame False {
              }
              frame True {
                n159 = property on="stop all" class="Bool (strict)"("DisabledEnum"=2) -> ()  [unwired: 2 in, 2 out]
              }
            }
          }
          event "Board select\n1: board 1\n2: board 2\n3: both boards": Value Change {
            # "selecting number of cams"
            n160 = event-data() -> ()  [unwired: 1 in, 6 out]
            n161 = global read "Globals.vi" "boards"() -> (w144:u32)
            n162 = case shown="2" w144 {
              frame 0, Default {
              }
              frame 2 {
                n163 = global write "Globals.vi" "board_sel"("Board select\n1: board 1\n2: board 2\n3: both boards") -> ()
              }
            }
          }
          event "continuous": Value Change {
            # "setting continuos mode"
            n164 = event-data() -> ()  [unwired: 1 in, 6 out]
            n165 = case shown="True" "continuous" {
              tunnel: [u8 0 u8 1] -> w146
              frame False {
              }
              frame True {
              }
            }
            n166 = call "contFFLoop.vi"("Numeric"=w146) -> ()  [unwired: 1 in]
          }
          event "alloc mem": Value Change {
            w154 = 0
            # "update params"
            # "Setup DMA"
            n167 = event-data() -> ()  [unwired: 1 in, 6 out]
            n168 = global read "Globals.vi" "CAMCNT"() -> (w153:u32)
            n169 = global read "Globals.vi" "nob"() -> (w151:u32)
            n170 = global read "Globals.vi" "nos"() -> (w152:u32)
            n171 = To Unsigned Long Integer(number=w153) -> (unsigned 32bit integer=w150:u32)
            n172 = global read "Globals.vi" "boards"() -> (w157:u32)
            n173 = case shown="2" w157 {
              selector: w157 -> [_ w159]
              tunnel: w152 -> [_ w160]
              tunnel: w151 -> [_ w161]
              tunnel: w150 -> [_ w158]
              frame 1, Default {
              }
              frame 2 {
                # "Setup DMA"
                n174 = call "SetupDMA_thread.vi"("camcnt"=w158, "blocks"=w161, "nos"=w160, "Drv"=w159) -> ()  [unwired: 1 in]
              }
            }
            n175 = call "SetupDMA_thread.vi"("camcnt"=w150, "blocks"=w151, "nos"=w152, "Drv"=u32 1) -> ()  [unwired: 1 in]
            n176 = property on="exposuretime[ms]" class="DigNum (strict)"() -> ("Value"=w156:dbl)  [unwired: 2 in, 2 out]
            n177 = property on="exposuretime[ms]" class="DigNum (strict)"("Val(Sgnl)"=w156) -> ()  [unwired: 2 in, 2 out]
            n178 = property on="continuous" class="Bool (strict)"("DisabledEnum"=w154) -> ()  [unwired: 2 in, 2 out]
            n179 = property on="block" class="Slide (strict)"("DisabledEnum"=w154) -> ()  [unwired: 2 in, 2 out]
            n180 = property on="sample" class="Slide (strict)"("DisabledEnum"=w154) -> ()  [unwired: 2 in, 2 out]
            n181 = property on="start" class="Bool (strict)"("DisabledEnum"=w154) -> ()  [unwired: 2 in, 2 out]
          }
          event "start": Mouse Down {
            # "start measurement"
            # "only 1st PCI board is used for ext. trig."
            # "ext. block trig\n0: internal: Space\n1: PCI \"I\"\n2: S1\n3: S2"
            # "block trigger 0/1\n0: internal -> next block is started immediately \n1: external -> each block has an own trigger"
            n182 = event-data() -> ()  [unwired: 1 in, 8 out]
            n183 = global read "Globals.vi" "exp time"() -> (w168:dbl)
            n184 = Multiply(x=1000.0, y=w168) -> (x*y=w170:dbl)
            n185 = global read "Globals.vi" "board_sel"() -> (w164:u8)
            n186 = To Unsigned Long Integer(number=w170) -> (unsigned 32bit integer=w166:u32)
            n187 = case shown="True" "extTrig" {
              tunnel: [u8 0 u8 1] -> w163
              frame False {
              }
              frame True {
              }
            }
            n188 = call "ReadFFLoop_thread.vi"("blocktrigger"=u8 0, "btrig_ch"=u8 0, "ExtTrig"=w163, "cam_sel"=w164, "exptus"=w166) -> ()  [unwired: 1 in]
          }
          event "sample", "block": Value Change {
            w189 = u32 1
            # "when selecting a value\nbigger than possible\nnos or nob, a dummy \nvalue \"1\" is chosen\n\nTODO:\ninsert error handling\nwith lower values than 1"
            # "display"
            n189 = event-data() -> ()  [unwired: 1 in, 6 out]
            n190 = global read "Globals.vi" "boards"() -> (w190:u32)
            n191 = global read "Globals.vi" "nob"() -> (w181:u32)
            n192 = global read "Globals.vi" "nos"() -> (w188:u32)
            n193 = Greater Or Equal?(x=w181, y="block") -> (x >= y?=w184:bool)
            n194 = Greater Or Equal?(x=w188, y="sample") -> (x >= y?=w187:bool)
            n195 = case shown="True" w184 {
              tunnel: [u32 1 w205] -> w183
              tunnel: "block" -> [_ w205]
              frame False {
                n196 = call "Display Message to User"() -> ()  [unwired: 10 in, 2 out]
              }
              frame True {
              }
            }
            n197 = case shown="False" w187 {
              tunnel: [u32 1 w207] -> w186
              tunnel: "sample" -> [_ w207]
              frame False {
                n198 = call "Display Message to User2"() -> ()  [unwired: 10 in, 2 out]
              }
              frame True {
              }
            }
            n199 = global read "Globals.vi" "CAMCNT"() -> (w174:u32)
            n200 = global read "Globals.vi" "PIXEL"() -> (w178:u32)
            n201 = Subtract(x=w186, y=w189) -> (x-y=w175:u32)
            n202 = Subtract(x=w183, y=w189) -> (x-y=w176:u32)
            n203 = case shown="2" w190 {
              selector: w190 -> [_ w212]
              tunnel: w175 -> [_ w213]
              tunnel: w176 -> [_ w210]
              frame 0, Default {
              }
              frame 2 {
                n204 = global read "Globals.vi" "PIXEL"() -> (w208:u32)
                n205 = To Long Integer(number=w208) -> (32bit integer=w209:i32)
                n206 = Initialize Array(u16 100, w209) -> (w215:u16[])
                n207 = call "ReturnFrame.vi"("Data Values In"=w215, "curr_nob"=w210, "curr_nos"=w213, "Drv"=w212) -> ("Data Values Out"=→"Signalverlaufgraph Board 2":u16[])  [unwired: 1 in]
              }
            }
            n208 = To Long Integer(number=w178) -> (32bit integer=w179:i32)
            n209 = Initialize Array(u16 100, w179) -> (w193:u16[])
            n210 = Multiply(x=w174, y=w175) -> (x*y=w173:u32)
            n211 = call "ReturnFrame.vi"("Data Values In"=w193, "curr_nob"=w176, "curr_nos"=w173, "Drv"=u32 1) -> ("Data Values Out"=→"Signalverlaufgraph":u16[])  [unwired: 1 in]
            n212 = global read "Globals.vi" "CAMCNT"() -> (w177:u32)
            n213 = case shown="2" w177 {
              tunnel: w176 -> [_ w197]
              tunnel: w173 -> [_ w195]
              frame 1, Default {
              }
              frame 2 {
                n214 = Add(x=w195, y=u32 1) -> (x+y=w196:u32)
                n215 = global read "Globals.vi" "PIXEL"() -> (w202:u32)
                n216 = To Long Integer(number=w202) -> (32bit integer=w201:i32)
                n217 = Initialize Array(u16 100, w201) -> (w198:u16[])
                n218 = call "ReturnFrame.vi"("Data Values In"=w198, "curr_nob"=w197, "curr_nos"=w196, "Drv"=u32 1) -> ("Data Values Out"=→"Signalverlaufgraph Cam 2":u16[])  [unwired: 1 in]
              }
            }
          }
          event "no.of samples (nos)", "no.of blocks (nob)\npress enter", "exposuretime[ms]": Value Change {
            # "calculation of MB RAM an SEC and setting scale max"
            # "MB"
            # "ushort"
            n219 = event-data() -> ()  [unwired: 1 in, 7 out]
            n220 = global read "Globals.vi" "PIXEL"() -> (w241:u32)
            n221 = Multiply(x="no.of samples (nos)", y=w241) -> (x*y=w239:u32)
            n222 = Multiply(x=w239, y=u32 2) -> (x*y=w219:u32)
            n223 = global read "Globals.vi" "boards"() -> (w240:u32)
            n224 = global read "Globals.vi" "CAMCNT"() -> (w218:u32)
            n225 = global read "Globals.vi" "nos"() -> (w223:u32)
            n226 = global read "Globals.vi" "nob"() -> (w221:u32)
            n227 = To Unsigned Long Integer(number=w218) -> (unsigned 32bit integer=w217:u32)
            n228 = Multiply(x=w217, y=w219) -> (x*y=w216:u32)
            n229 = Multiply(x=w216, y=w240) -> (x*y=w229:u32)
            n230 = To Double Precision Float(number=w229) -> (double precision float=w228:dbl)
            n231 = To Double Precision Float(number=w223) -> (double precision float=w222:dbl)
            n232 = Divide(x=w228, y=1048576.0) -> (x/y=w231:dbl)
            n233 = To Double Precision Float(number=w221) -> (double precision float=w220:dbl)
            n234 = To Double Precision Float(number="no.of blocks (nob)\npress enter") -> (double precision float=w226:dbl)
            n235 = property on="sample" class="Slide (strict)"("Scale.Maximum"=w222) -> ()  [unwired: 2 in, 2 out]
            n236 = property on="block" class="Slide (strict)"("Scale.Maximum"=w220) -> ()  [unwired: 2 in, 2 out]
            n237 = Multiply(x=w231, y=w226) -> (x*y=→"MB RAM":dbl)
            n238 = global write "Globals.vi" "nos"("no.of samples (nos)") -> ()
            n239 = Multiply(x="no.of samples (nos)", y="no.of blocks (nob)\npress enter") -> (x*y=w224:u32)
            n240 = global write "Globals.vi" "nob"("no.of blocks (nob)\npress enter") -> ()
            n241 = To Double Precision Float(number=w224) -> (double precision float=w225:dbl)
            n242 = global write "Globals.vi" "exp time"("exposuretime[ms]") -> ()
            n243 = Multiply(x="exposuretime[ms]", y=w225) -> (x*y=w237:dbl)
            n244 = Divide(x=w237, y=1000.0) -> (x/y=→"SEC":dbl)
          }
          event "stop all": Value Change {
            # "exit"
            n245 = event-data() -> ()  [unwired: 1 in, 6 out]
            n246 = stacked-sequence {
              tunnel: [_ TRUE] -> w242
              frame #0 {
                n247 = call "FFStop.vi"() -> ()  [unwired: 1 in]
              }
              frame #1 {
                # "do not omit, or next call of driver will go wrong."
                n248 = call "Exit.vi"() -> ()  [unwired: 1 in]
              }
            }
          }
          event "rms_pixel": Value Change {
            # "one array with all values (except first 10)\nat index Pixel from all blocks"
            n249 = event-data() -> ()  [unwired: 1 in, 6 out]
            n250 = global read "Globals.vi" "nos"() -> (w248:u32)
            n251 = global read "Globals.vi" "nob"() -> (w249:u32)
            n252 = for {
              N: w249 -> [_]
              tunnel: w248 -> [w250]
              tunnel: [w252] -> w245 mode=concatenating
              i -> [w256]
              # "delete first 10 values"
              # "array of all values\nat index Pixel"
              n253 = To Long Integer(number=w250) -> (32bit integer=w251:i32)
              n254 = for {
                N: w251 -> [_]
                tunnel: w256 -> [w261]
                tunnel: [w265] -> w253 mode=indexing
                i -> [w263]
                # "use only value at index \"Pixel\""
                # "init array of size PIXEL\nwith value 100"
                n255 = global read "Globals.vi" "PIXEL"() -> (w257:u32)
                n256 = To Long Integer(number=w257) -> (32bit integer=w258:i32)
                n257 = To Unsigned Long Integer(number=w261) -> (unsigned 32bit integer=w262:u32)
                n258 = To Unsigned Long Integer(number=w263) -> (unsigned 32bit integer=w264:u32)
                n259 = Initialize Array(u16 100, w258) -> (w267:u16[])
                n260 = call "ReturnFrame.vi"("Data Values In"=w267, "curr_nob"=w262, "curr_nos"=w264, "Drv"=u32 1) -> ("Data Values Out"=w266:u16[])  [unwired: 1 in]
                n261 = To Long Integer(number="rms_pixel") -> (32bit integer=w259:i32)
                n262 = Index Array(array=w266, index=w259) -> (element=w265:u16)
              }
              n263 = Delete From Array(array=w253, length=10, index=0) -> (array with subset deleted=w252:u16[])  [unwired: 1 out]
            }
            n264 = To Double Precision Float(number=w245) -> (double precision float=w244:dbl[])
            n265 = call <vilib>:"Std Deviation and Variance.vi"("X"=w244) -> ("mean"=→"mean":dbl, "standard deviation"=→"tRMS":dbl)  [unwired: 1 in, 1 out]
          }
          event "ADC mode", "custom pattern: 14bits (hex)": Value Change {
            n266 = event-data() -> ()  [unwired: 1 in, 6 out]
            n267 = case shown="\"1\"" "ADC mode" {
              frame "1" {
                w294 = u8 38  # adadr (hex)
                w295 = u8 37  # adadr (hex)
                # "Custom Pattern"
                n268 = Number To Boolean Array(number="custom pattern: 14bits (hex)") -> (Boolean array=w293:bool[])
                n269 = Number To Boolean Array(number="custom pattern: 14bits (hex)") -> (Boolean array=w290:bool[])
                n270 = Number To Boolean Array(number=fxp<+,12,12> 4.0) -> (Boolean array=w285:bool[])
                n271 = Array Subset(array=w293, index=0, length=12) -> (w275:bool[])
                n272 = Array Subset(array=w290, index=12, length=2) -> (w286:bool[])
                n273 = Insert Into Array(array=w285, index=0, new element=w286) -> (w283:bool[])
                n274 = Number To Boolean Array(number=fxp<+,4,4> 0.0) -> (Boolean array=w276:bool[])
                n275 = Boolean Array To Number(Boolean array=w283) -> (number=w282:u32)
                n276 = Insert Into Array(array=w275, index=0, new element=w276) -> (w274:bool[])
                n277 = To Unsigned Word Integer(number=w282) -> (unsigned 16bit integer=w278:u16)
                "data adr  0x25" <- w278
                n278 = Boolean Array To Number(Boolean array=w274) -> (number=w279:u32)
                n279 = To Unsigned Word Integer(number=w279) -> (unsigned 16bit integer=w277:u16)
                "data adr  0x26" <- w277
                n280 = global read "Globals.vi" "maddr of ADC"() -> (w271:u8)
                n281 = global read "Globals.vi" "maddr of ADC"() -> (w272:u8)
                n282 = call "SendFLCam.vi"("madr"=w272, "data"=w278, "adadr"=w295) -> ()
                n283 = call "SendFLCam.vi"("madr"=w271, "data"=w277, "adadr"=w294) -> ()
                "custom pattern: 14bits (dec)" <- "custom pattern: 14bits (hex)"
              }
              frame "2" {
                w297 = u16 0  # data (hex)
                w298 = u16 64  # data (hex)
                w299 = u8 37  # adadr (hex)
                # "Ramp"
                n284 = global read "Globals.vi" "maddr of ADC"() -> (w296:u8)
                n285 = call "SendFLCam.vi"("madr"=w296, "data"=w298, "adadr"=w299) -> ()
                n286 = property on="data adr  0x26" class="DigNum (strict)"("Val(Sgnl)"=w297) -> ()  [unwired: 2 in, 2 out]
                n287 = property on="data adr  0x25" class="DigNum (strict)"("Val(Sgnl)"=w298) -> ()  [unwired: 2 in, 2 out]
              }
              frame "3" {
                w305 = u16 1  # data
                w306 = u8 0  # adadr (hex)
                w304 = u16 0  # data
                w307 = u8 38  # adadr (hex)
                w303 = u16 0  # data
                w308 = u8 37  # adadr (hex)
                # "Normal Mode"
                n288 = global read "Globals.vi" "maddr of ADC"() -> (w301:u8)
                n289 = global read "Globals.vi" "maddr of ADC"() -> (w302:u8)
                n290 = global read "Globals.vi" "maddr of ADC"() -> (w300:u8)
                n291 = call "SendFLCam.vi"("madr"=w301, "data"=w304, "adadr"=w307) -> ()
                n292 = call "SendFLCam.vi"("madr"=w302, "data"=w305, "adadr"=w306) -> ()
                n293 = call "SendFLCam.vi"("madr"=w300, "data"=w303, "adadr"=w308) -> ()
                n294 = property on="data adr  0x26" class="DigNum (strict)"("Val(Sgnl)"=w304) -> ()  [unwired: 2 in, 2 out]
                n295 = property on="data adr  0x25" class="DigNum (strict)"("Val(Sgnl)"=w303) -> ()  [unwired: 2 in, 2 out]
              }
            }
          }
          event "Offset ADC 4": Value Change {
            w313 = fxp<+,4,4> 0.0  # feature (hex)
            w312 = fxp<+,4,4> 0.0  # addr (hex)
            w310 = fxp<+,4,4> 3.0  # ctrl (hex)
            # "Register CHA"
            # "ctrl: write and update DAC register"
            n296 = event-data() -> ()  [unwired: 1 in, 6 out]
            n297 = To Unsigned Byte Integer(number=w313) -> (unsigned 8bit integer=w314:u8)
            n298 = To Unsigned Byte Integer(number=w312) -> (unsigned 8bit integer=w315:u8)
            n299 = To Unsigned Byte Integer(number=w310) -> (unsigned 8bit integer=w311:u8)
            n300 = call "SendFLCam_DAC.vi"("ctrl"=w311, "feature"=w314, "data"="Offset ADC 4", "addr"=w315) -> ()
          }
          event "Offset ADC 5": Value Change {
            w319 = fxp<+,4,4> 0.0  # feature (hex)
            w318 = fxp<+,4,4> 1.0  # addr (hex)
            w316 = fxp<+,4,4> 3.0  # ctrl (hex)
            # "Register CHB"
            # "ctrl: write and update DAC register"
            n301 = event-data() -> ()  [unwired: 1 in, 6 out]
            n302 = To Unsigned Byte Integer(number=w319) -> (unsigned 8bit integer=w320:u8)
            n303 = To Unsigned Byte Integer(number=w318) -> (unsigned 8bit integer=w321:u8)
            n304 = To Unsigned Byte Integer(number=w316) -> (unsigned 8bit integer=w317:u8)
            n305 = call "SendFLCam_DAC.vi"("ctrl"=w317, "feature"=w320, "data"="Offset ADC 5", "addr"=w321) -> ()
          }
          event "Offset ADC 1": Value Change {
            w326 = fxp<+,4,4> 0.0  # feature (hex)
            w325 = fxp<+,4,4> 2.0  # addr (hex)
            w323 = fxp<+,4,4> 3.0  # ctrl (hex)
            # "Register CHC"
            # "ctrl: write and update DAC register"
            n306 = event-data() -> ()  [unwired: 1 in, 6 out]
            n307 = To Unsigned Byte Integer(number=w326) -> (unsigned 8bit integer=w327:u8)
            n308 = To Unsigned Byte Integer(number=w325) -> (unsigned 8bit integer=w328:u8)
            n309 = To Unsigned Byte Integer(number=w323) -> (unsigned 8bit integer=w324:u8)
            n310 = call "SendFLCam_DAC.vi"("ctrl"=w324, "feature"=w327, "data"="Offset ADC 1", "addr"=w328) -> ()
          }
          event "Offset ADC 6": Value Change {
            w333 = fxp<+,4,4> 0.0  # feature (hex)
            w332 = fxp<+,4,4> 3.0  # addr (hex)
            w330 = fxp<+,4,4> 3.0  # ctrl (hex)
            # "Register CHD"
            # "ctrl: write and update DAC register"
            n311 = event-data() -> ()  [unwired: 1 in, 6 out]
            n312 = To Unsigned Byte Integer(number=w333) -> (unsigned 8bit integer=w334:u8)
            n313 = To Unsigned Byte Integer(number=w332) -> (unsigned 8bit integer=w335:u8)
            n314 = To Unsigned Byte Integer(number=w330) -> (unsigned 8bit integer=w331:u8)
            n315 = call "SendFLCam_DAC.vi"("ctrl"=w331, "feature"=w334, "data"="Offset ADC 6", "addr"=w335) -> ()
          }
          event "Offset ADC 2": Value Change {
            w340 = fxp<+,4,4> 0.0  # feature (hex)
            w339 = fxp<+,4,4> 4.0  # addr (hex)
            w337 = fxp<+,4,4> 3.0  # ctrl (hex)
            # "Register CHE"
            # "ctrl: write and update DAC register"
            n316 = event-data() -> ()  [unwired: 1 in, 6 out]
            n317 = To Unsigned Byte Integer(number=w340) -> (unsigned 8bit integer=w341:u8)
            n318 = To Unsigned Byte Integer(number=w339) -> (unsigned 8bit integer=w342:u8)
            n319 = To Unsigned Byte Integer(number=w337) -> (unsigned 8bit integer=w338:u8)
            n320 = call "SendFLCam_DAC.vi"("ctrl"=w338, "feature"=w341, "data"="Offset ADC 2", "addr"=w342) -> ()
          }
          event "Offset ADC 7": Value Change {
            w347 = fxp<+,4,4> 0.0  # feature (hex)
            w346 = fxp<+,4,4> 5.0  # addr (hex)
            w344 = fxp<+,4,4> 3.0  # ctrl (hex)
            # "Register CHF"
            # "ctrl: write and update DAC register"
            n321 = event-data() -> ()  [unwired: 1 in, 6 out]
            n322 = To Unsigned Byte Integer(number=w347) -> (unsigned 8bit integer=w348:u8)
            n323 = To Unsigned Byte Integer(number=w346) -> (unsigned 8bit integer=w349:u8)
            n324 = To Unsigned Byte Integer(number=w344) -> (unsigned 8bit integer=w345:u8)
            n325 = call "SendFLCam_DAC.vi"("ctrl"=w345, "feature"=w348, "data"="Offset ADC 7", "addr"=w349) -> ()
          }
          event "Offset ADC 3": Value Change {
            w354 = fxp<+,4,4> 0.0  # feature (hex)
            w353 = fxp<+,4,4> 6.0  # addr (hex)
            w351 = fxp<+,4,4> 3.0  # ctrl (hex)
            # "Register CHG"
            # "ctrl: write and update DAC register"
            n326 = event-data() -> ()  [unwired: 1 in, 6 out]
            n327 = To Unsigned Byte Integer(number=w354) -> (unsigned 8bit integer=w355:u8)
            n328 = To Unsigned Byte Integer(number=w353) -> (unsigned 8bit integer=w356:u8)
            n329 = To Unsigned Byte Integer(number=w351) -> (unsigned 8bit integer=w352:u8)
            n330 = call "SendFLCam_DAC.vi"("ctrl"=w352, "feature"=w355, "data"="Offset ADC 3", "addr"=w356) -> ()
          }
          event "Offset ADC 8": Value Change {
            w361 = fxp<+,4,4> 0.0  # feature (hex)
            w360 = fxp<+,4,4> 7.0  # addr (hex)
            w358 = fxp<+,4,4> 3.0  # ctrl (hex)
            # "Register CHH"
            # "ctrl: write and update DAC register"
            n331 = event-data() -> ()  [unwired: 1 in, 6 out]
            n332 = To Unsigned Byte Integer(number=w361) -> (unsigned 8bit integer=w362:u8)
            n333 = To Unsigned Byte Integer(number=w360) -> (unsigned 8bit integer=w363:u8)
            n334 = To Unsigned Byte Integer(number=w358) -> (unsigned 8bit integer=w359:u8)
            n335 = call "SendFLCam_DAC.vi"("ctrl"=w359, "feature"=w362, "data"="Offset ADC 8", "addr"=w363) -> ()
          }
          event "send all": Value Change {
            n336 = event-data() -> ()  [unwired: 1 in, 6 out]
            n337 = property on="Offset ADC 1" class="DigNum (strict)"() -> ("Value"=w365:u16)  [unwired: 2 in, 2 out]
            n338 = property on="Offset ADC 4" class="DigNum (strict)"() -> ("Value"=w368:u16)  [unwired: 2 in, 2 out]
            n339 = property on="Offset ADC 2" class="DigNum (strict)"() -> ("Value"=w366:u16)  [unwired: 2 in, 2 out]
            n340 = property on="Offset ADC 3" class="DigNum (strict)"() -> ("Value"=w367:u16)  [unwired: 2 in, 2 out]
            n341 = property on="Offset ADC 1" class="DigNum (strict)"("Val(Sgnl)"=w365) -> ()  [unwired: 2 in, 2 out]
            n342 = property on="Offset ADC 4" class="DigNum (strict)"("Val(Sgnl)"=w368) -> ()  [unwired: 2 in, 2 out]
            n343 = property on="Offset ADC 2" class="DigNum (strict)"("Val(Sgnl)"=w366) -> ()  [unwired: 2 in, 2 out]
            n344 = property on="Offset ADC 3" class="DigNum (strict)"("Val(Sgnl)"=w367) -> ()  [unwired: 2 in, 2 out]
            n345 = property on="Offset ADC 8" class="DigNum (strict)"() -> ("Value"=w372:u16)  [unwired: 2 in, 2 out]
            n346 = property on="Offset ADC 5" class="DigNum (strict)"() -> ("Value"=w369:u16)  [unwired: 2 in, 2 out]
            n347 = property on="Offset ADC 7" class="DigNum (strict)"() -> ("Value"=w371:u16)  [unwired: 2 in, 2 out]
            n348 = property on="Offset ADC 6" class="DigNum (strict)"() -> ("Value"=w370:u16)  [unwired: 2 in, 2 out]
            n349 = property on="Offset ADC 8" class="DigNum (strict)"("Val(Sgnl)"=w372) -> ()  [unwired: 2 in, 2 out]
            n350 = property on="Offset ADC 5" class="DigNum (strict)"("Val(Sgnl)"=w369) -> ()  [unwired: 2 in, 2 out]
            n351 = property on="Offset ADC 7" class="DigNum (strict)"("Val(Sgnl)"=w371) -> ()  [unwired: 2 in, 2 out]
            n352 = property on="Offset ADC 6" class="DigNum (strict)"("Val(Sgnl)"=w370) -> ()  [unwired: 2 in, 2 out]
          }
        }
      }
    }
  }
  n353 = property on="sample" class="Slide (strict)"("DisabledEnum"=w1) -> ()  [unwired: 2 in, 2 out]
  n354 = property on="start" class="Bool (strict)"("DisabledEnum"=w1) -> ()  [unwired: 2 in, 2 out]
  n355 = property on="block" class="Slide (strict)"("DisabledEnum"=w1) -> ()  [unwired: 2 in, 2 out]
